vi "From JSON.vi"(8 "error in":errorcluster, 10 "JSON Config":path, 11 "object in":refnum<class "Camera Imaqdx CFG.lvclass">) -> (0 "error out":errorcluster, 3 "object out":refnum<class "Camera Imaqdx CFG.lvclass">)   [LabVIEW 2023, in "HAL.lvlib" / "Camera Imaqdx CFG.lvclass"]
uses:
  Camera Imaqdx CFG.lvclass
  Camera Imaqdx CFG.lvclass/Camera Imaqdx CFG.ctl
  <vilib>/ErrorRing/Error Ring.xnode
  Configuration Base/Configuration Base.lvclass
  52c82fbc-93b2-4944-a492-f162528988d3.vi
  <vilib>/Utility/error.llb/Error Cluster From Error Code.vi
  D:/git/HAL/Configuration Base/Configuration Base.lvclass
  D:/git/HAL/Interfaces/IConfigure/IConfigure.lvclass
  D:/git/HAL/Camera Imaqdx/Configuration/Camera Imaqdx CFG.lvclass
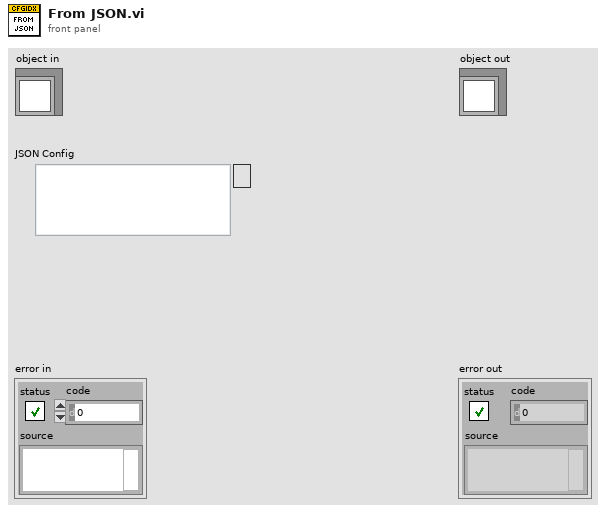
[diagram p1: front panel]
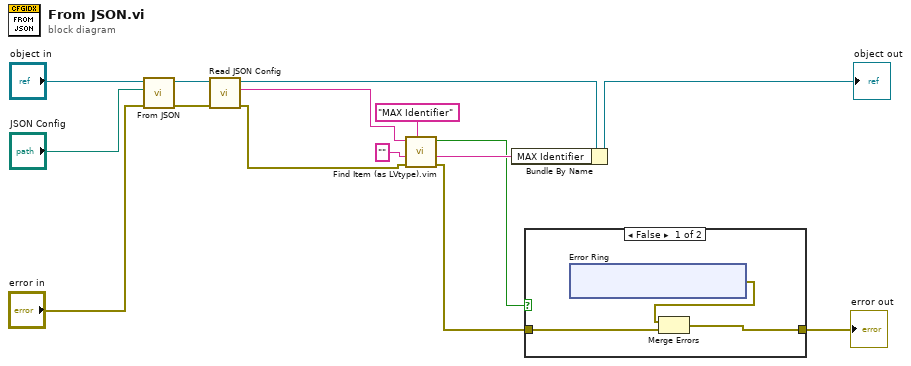
[diagram p0: block diagram]
diagram:
  n1 = call-parent "From JSON.vi"("error in (no error)"="error in", "JSON Config"="JSON Config", "object in"="object in") -> ("error out"=w9:errorcluster, "object out"=w6:refnum<class "Camera Imaqdx CFG.lvclass">)  [unwired: 7 in]
  n2 = call "Read JSON Config.vi"("error in"=w9, "object in"=w6) -> ("error out"=w7:errorcluster, "<JSON>Config"=w4:string, "object out"=w2:refnum<class "Camera Imaqdx CFG.lvclass">)  [unwired: 7 in]
  n3 = call "Find Item (as LVtype).vim"("$Path or Item Name"="MAX Identifier", "error in (no error)"=w7, "Data Type and Default Value"="", "JSON"=w4) -> ("error out"=w11:errorcluster, "Data"=w13:string, "Found"=w12:bool)  [unwired: 4 in, 1 out]
  n4 = Bundle By Name(cluster=w2, "MAX Identifier"=w13) -> (→"object out":refnum<class "Camera Imaqdx CFG.lvclass">)
  n5 = case shown="False" w12 {
    tunnel: w11 -> [w18 w24]
    tunnel: [w16 w24] -> w14
    frame False {
      n6 = xnode "Error Ring"() -> ("error out"=w17:errorcluster)
      n7 = Merge Errors(w17, w18) -> (w16:errorcluster)
    }
    frame True {
    }
  }
  "error out" <- w14
